vi "Part 1.vi"(11 "Input":string) -> (3 "Output":i64)   [LabVIEW 2021]
uses:
  <userlib>/_OpenG.lib/string/string.llb/Convert EOLs (String)__ogtk.vi
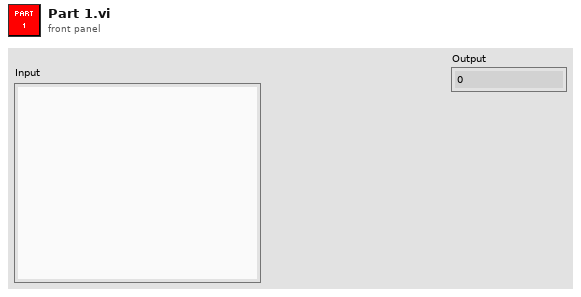
[diagram p1: front panel]
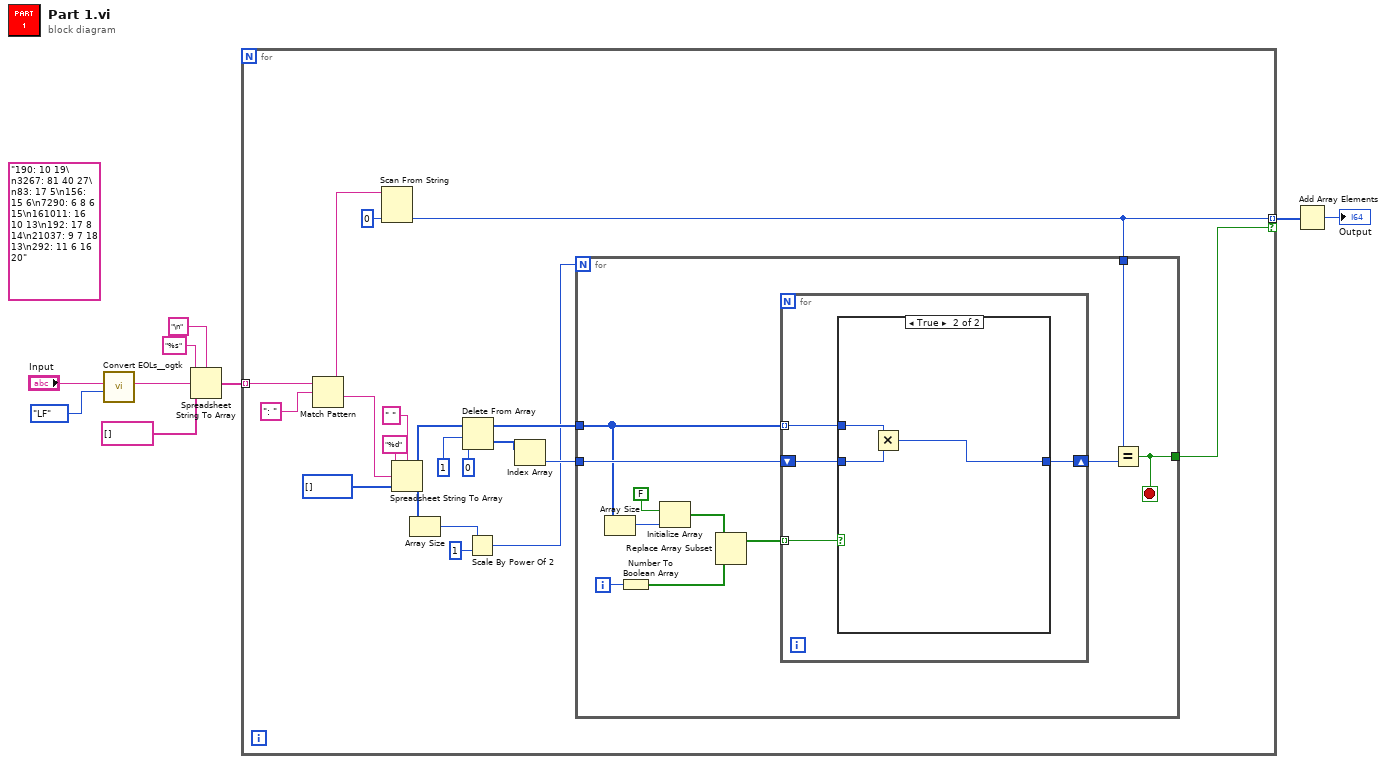
[diagram p0: block diagram]
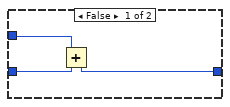
[diagram p2: hidden frame]
diagram:
  (unwired) "190: 10 19\n3267: 81 40 27\n83: 17 5\n156: 15 6\n7290: 6 8 6 15\n161011: 16 10 13\n192: 17 8 14\n21037: 9 7 18 13\n292: 11 6 16 20"
  n1 = call-poly <userlib>:"Convert EOLs__ogtk.vi"("Convert to:"=enum16{"CR", "LF", "CRLF"}."LF", "String in"="Input") -> ("String out"=w6:string)  [unwired: 9 in]
  n2 = Spreadsheet String To Array(delimiter (Tab)="\n", format string="%s", spreadsheet string=w6, array type (2D Dbl)=string[] []) -> (array=w4:string[])
  n3 = for {
    tunnel: w4 -> [w28] mode=indexing
    tunnel: [w14] -> w3 mode=indexing if=w13
    n4 = Match Pattern(string=w28, regular expression=": " ("delimiter (Tab)")) -> (before substring=w26:string, after substring=w25:string)  [unwired: 1 in, 2 out]
    n5 = Scan From String(input string=w26, default 1=i64 0) -> (output 1=w14:i64)  [unwired: 3 in, 3 out]
    n6 = Spreadsheet String To Array(delimiter (Tab)=" ", format string="%d", spreadsheet string=w25, array type (2D Dbl)=i64[] []) -> (array=w20:i64[])
    n7 = Array Size(array=w20) -> (size(s)=w12:i32)
    n8 = Delete From Array(array=w20, length=1, index=0) -> (deleted portion=w16:i64[], array with subset deleted=w17:i64[])
    n9 = Scale By Power Of 2(n=w12, x=1) -> (x*2^n=w10:i32)
    n10 = Index Array(array=w16) -> (element=w15:i64)  [unwired: 1 in]
    n11 = for {
      N: w10 -> [_]
      tunnel: w17 -> [w34]
      tunnel: w15 -> [w39]
      tunnel: w14 -> [w37]
      tunnel: [w36] -> w13
      i -> [w35]
      stop <- w36 stop-if-true
      n12 = Array Size(array=w34) -> (size(s)=w33:i32)
      n13 = Number To Boolean Array(number=w35) -> (Boolean array=w30:bool[])
      n14 = Initialize Array(FALSE, w33) -> (w31:bool[])
      n15 = Replace Array Subset(array=w31, new element=w30) -> (w29:bool[])  [unwired: 1 in]
      n16 = for {
        tunnel: w34 -> [w41] mode=indexing
        shift-right: [w40] -> w38
        shift-left: w39 -> [w42]
        tunnel: w29 -> [w43] mode=indexing
        n17 = case shown="True" w43 {
          tunnel: w42 -> [w46 w49]
          tunnel: w41 -> [w45 w48]
          tunnel: [w44 w47] -> w40
          frame False {
            n18 = Add(x=w45, y=w46) -> (x+y=w44:i64)
          }
          frame True {
            n19 = Multiply(x=w48, y=w49) -> (x*y=w47:i64)
          }
        }
      }
      n20 = Equal?(x=w37, y=w38) -> (x = y?=w36:bool)
    }
  }
  n21 = Add Array Elements(numeric array=w3) -> (sum=→"Output":i64)
